vi "MovingTime.vi"(8 "error in":errorcluster, 9 "Acc (mm/s^2)":dbl=1.5, 10 "MaxV (mm/s)":dbl=2.5, 11 "Distance (mm)":dbl=0.1 format="%#_13g") -> (0 "error out":errorcluster, 3 "time (s)":dbl)   [LabVIEW 2014]
doc: "This VI is used to calculate the moving time of the stage. The shape of the velocity vs. time graph could be a Triangle or a Trapezoid."
panel:
  # "This VI is used to calculate the moving time of the stage. The shape of the velocity vs. time graph could be  a Triangle or a Trapezoid.\n\nIf D<0.5*(v/a)*v*2, D=0.5*a*(t/2)^2*2, so t=sqrt(4*D/a)\n\nIf D>0.5*(v/a)*v*2, D=v^2/a+v*(t-2*v/a), so t=(D-v^2/a)/v+2*v/a\n\nD.1.3 Velocity Profiles\nTo prevent the motor from stalling, it must be ramped up gradually to its maximum velocity. Certain limits to velocity and acceleration result from the torque and speed limits of the motor, and the inertia and friction of the parts it drives. \nThe motion employed is described by a trapezoidal velocity profile, reflecting the shape of the velocity vs. time graph (see Fig. D.2.), thereby driving the stage to its destination as quickly as possible, without causing it to stall or lose steps.\nThe stage is ramped at acceleration ‘a’ to a maximum velocity ‘v’. As the destination is approached, the stage is decelerated at ‘a’ so that the final position is approached slowly in a controlled manner."
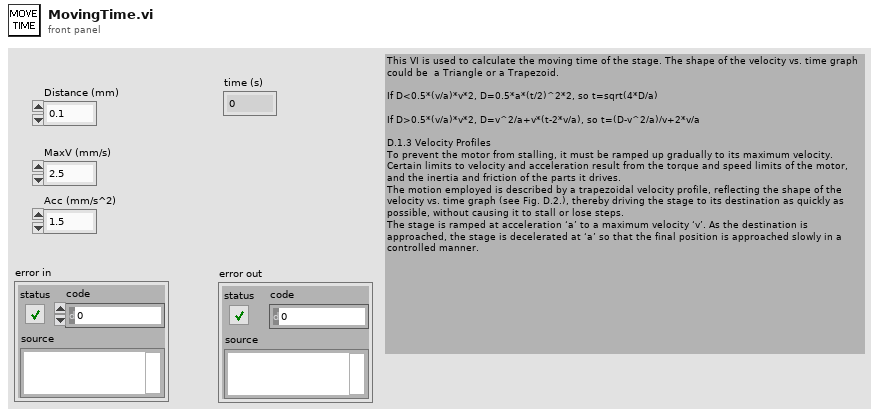
[diagram p1: front panel]
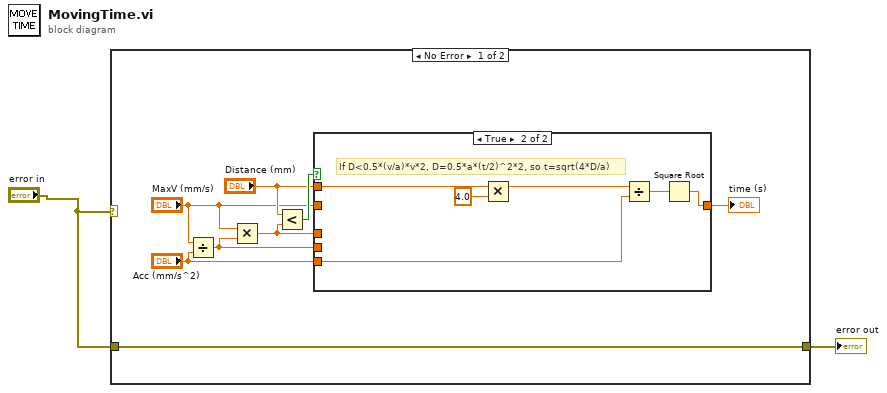
[diagram p0: block diagram]
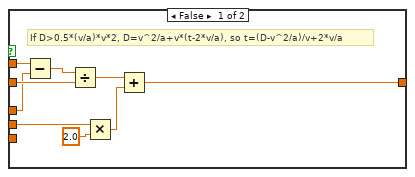
[diagram p2: hidden frame]
diagram:
  n1 = case shown="No Error" "error in" {
    tunnel: "error in" -> [w3 w26]
    tunnel: [w3 w26] -> w1
    frame No Error {
      n2 = Divide(x="MaxV (mm/s)", y="Acc (mm/s^2)") -> (x/y=w4:dbl)
      n3 = Multiply(x="MaxV (mm/s)", y=w4) -> (x*y=w5:dbl)
      n4 = Less?(x="Distance (mm)", y=w5) -> (x < y?=w10:bool)
      n5 = case shown="True" w10 {
        tunnel: "Distance (mm)" -> [w19 w22]
        tunnel: "Acc (mm/s^2)" -> [_ w24]
        tunnel: [w11 w25] -> w7
        tunnel: "MaxV (mm/s)" -> [w17 _]
        tunnel: w5 -> [w16 _]
        tunnel: w4 -> [w14 _]
        frame False {
          # "If D>0.5*(v/a)*v*2, D=v^2/a+v*(t-2*v/a), so t=(D-v^2/a)/v+2*v/a"
          n6 = Subtract(x=w19, y=w16) -> (x-y=w18:dbl)
          n7 = Divide(x=w18, y=w17) -> (x/y=w15:dbl)
          n8 = Multiply(x=w14, y=2.0) -> (x*y=w12:dbl)
          n9 = Add(x=w15, y=w12) -> (x+y=w11:dbl)
        }
        frame True {
          # "If D<0.5*(v/a)*v*2, D=0.5*a*(t/2)^2*2, so t=sqrt(4*D/a)"
          n10 = Multiply(x=w22, y=4.0) -> (x*y=w21:dbl)
          n11 = Divide(x=w21, y=w24) -> (x/y=w23:dbl)
          n12 = Square Root(x=w23) -> (sqrt(x)=w25:dbl)
        }
      }
      "time (s)" <- w7
    }
    frame Error {
    }
  }
  "error out" <- w1
